vi "LVClass_SlopesPostProcessList AddProcessor_Substractor.vi"(0 "SlopesPostProcessorList in":refnum<class "SlopesPostProcessorList.lvclass">, 5 "Position":i32, 7 "HasoSlopes.lvclass":refnum<class "HasoSlopes.lvclass">, 9 "Comment":string, 11 "error in (no error)":errorcluster) -> (4 "SlopesPostProcessorList out":refnum<class "SlopesPostProcessorList.lvclass">, 15 "error out":errorcluster)   [LabVIEW 2020, in "SlopesPostProcessorList.lvclass"]
doc: "Insert a Substractor processor.\n\n--------------------------------------------------------------------------------\n\n<B>SlopesPostProcessorListIn </B> : SlopesPostProcessorList object.\n<B>SlopesPostProcessorListOut </B> : SlopesPostProcessorList object.\n<B>position </B> : Position of the processor in the SlopesPostProcessorList.\n<B>comment </B> : Comments.\n<B>HasoSlopes </B> : HasoSlopes to set in the processor.\n<B>ErrorIn </B> : Error\n<B>ErrorOut </B> : Error\n\n--------------------------------------------------------------------------------"
uses:
  SlopesPostProcessorList.lvclass
  HasoSlopes/HasoSlopes.lvclass
  SlopesPostProcessorList.lvclass/SlopesPostProcessorList.ctl
  HasoSlopes/LVClass_HasoSlopes Read HasoSlopes _ property.vi
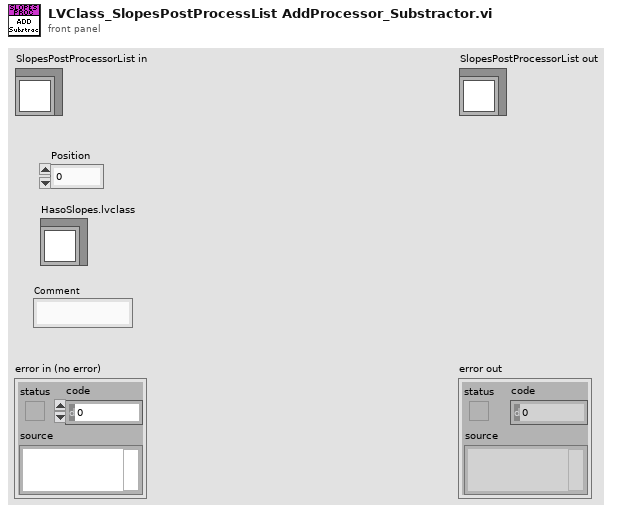
[diagram p1: front panel]
types:
  T1 = typedef "ClassID.ctl" = i64
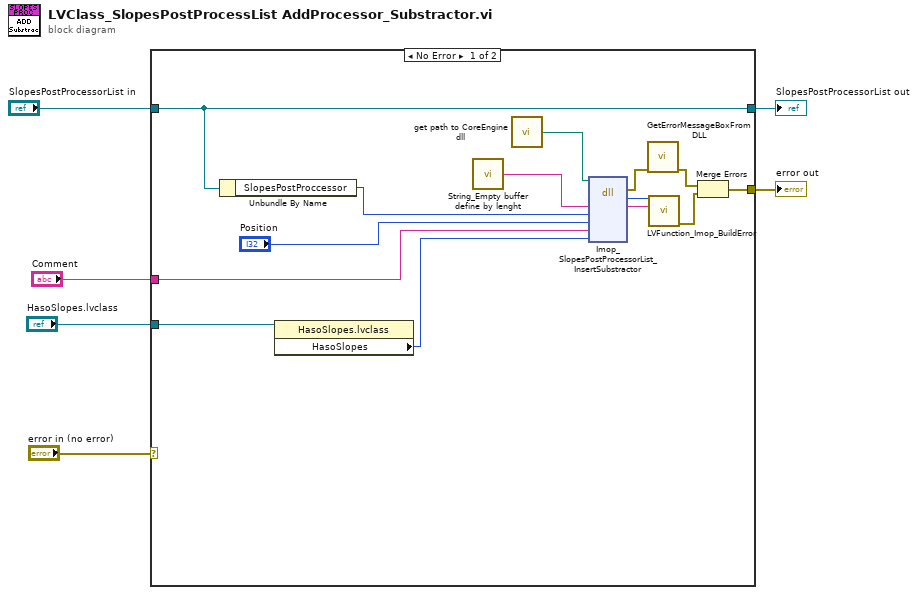
[diagram p0: block diagram]
diagram:
  n1 = case shown="No Error" "error in (no error)" {
    selector: "error in (no error)" -> [_ w22]
    tunnel: [w8 w22] -> w5
    tunnel: [w12 w21] -> w3
    tunnel: "SlopesPostProcessorList in" -> [w12 w21]
    tunnel: "HasoSlopes.lvclass" -> [w14 _]
    tunnel: "Comment" -> [w7 _]
    frame No Error {
      n2 = Unbundle By Name(w12) -> ("SlopesPostProccessor"=w11:T1)
      n3 = property class="HasoSlopes.lvclass"(reference=w14) -> ("HasoSlopes"=w13:T1)  [unwired: 1 in, 2 out]
      n4 = call "String_Empty buffer define by lenght.vi"() -> ("Empty buffer"=w20:string)  [unwired: 1 in]
      n5 = call "get path to CoreEngine dll.vi"() -> ("path to wavekit library"=w17:path)  [unwired: 14 in, 1 out]
      n6 = dll-call lib="D:/soft/HASO_v3/SVN_trunk/ImOpCoreEngine4_LV2011/DLLs/c_interface_vc100.dll" fn="Imop_SlopesPostProcessorList_InsertSubstractor"(path in=w17, "message"=w20, "objet"=w11, "Position"="Position", "Comment"=w7, "HasoSlopes"=w13) -> (error out=w16:errorcluster, "return type"=w18:i32, "message"=w19:string)  [unwired: 6 in, 1 out]
      n7 = call "GetErrorMessageBoxFromDLL.vi"("error IN"=w16) -> ("error OUT"=w10:errorcluster)  [unwired: 10 in]
      n8 = call "LVFunction_Imop_BuildError.vi"("code"=w18, "String to Prepend to source (\"\")"=w19) -> ("error out"=w9:errorcluster)  [unwired: 13 in]
      n9 = Merge Errors(w10, w9) -> (w8:errorcluster)
    }
    frame Error {
    }
  }
  "error out" <- w5
  "SlopesPostProcessorList out" <- w3
